vi "ModelProject_backup.vi"() -> ()   [LabVIEW 2011]
uses:
  <vilib>/Simulation/Scripting/Companion Diagram/SimConfigNode/SimParams.ctl
  <vilib>/Simulation/Scripting/Companion Diagram/SimConfigNode/_simSolvers.ctl
  <vilib>/Simulation/Implementation/Shared/SIMSCR Execution Mode.ctl
  <vilib>/Simulation/Param Hierarchy/Typedefs/SIMPH Param Control Actions.ctl
  <vilib>/Simulation/Implementation/Shared/SIM limit type.ctl
  <vilib>/Simulation/Implementation/Shared/NILVSim_FinalizeModel.vi
  <vilib>/Simulation/SignalDisplay/Implementation/NILVSim Buffer XY Graph.llb/SIM Buffer XY Graph (scalar).vi
  <vilib>/Simulation/Utility/Implementation/SIM Time.vi
  <vilib>/Simulation/SignalDisplay/Implementation/NILVSim Time Waveform.llb/SIM Time Waveform (scalar).vi
  <vilib>/Simulation/ContinuousLinear/Implementation/NILVSim Integrator new.llb/SIM Integrator distributor (scalar).vi
  <vilib>/Simulation/ContinuousLinear/Implementation/NILVSim Integrator new.llb/SIM Integrator collector (scalar).vi
  <vilib>/Simulation/ContinuousLinear/Implementation/NILVSim Transfer Function.llb/SIM Transfer Function Collector (SISO).vi
  <vilib>/Simulation/ContinuousLinear/Implementation/NILVSim Transfer Function.llb/SIM Transfer Function Distributor (SISO).vi
  <vilib>/Simulation/ContinuousLinear/Implementation/NILVSim State Space.llb/SIM State Space Distributor (SISO CD).vi
  <vilib>/Simulation/ContinuousLinear/Implementation/NILVSim State Space.llb/SIM State Space Collector (SISO CD).vi
  <vilib>/Simulation/Implementation/Shared/SIM Is Init or Final Stage.vi
  <vilib>/Simulation/Implementation/Shared/NILVSim_Manager.vi
  <vilib>/Simulation/Implementation/Shared/NILVSim_ParamChanged.vi
  <vilib>/Simulation/SignalDisplay/Implementation/NILVSim Buffer XY Graph.llb/NILVSim Buffer XY Graph (core).vi
  <vilib>/Simulation/Implementation/Shared/SIM manage modulo counter.vi
  <vilib>/Simulation/Implementation/Shared/SIM Circular Buffer.llb/SIM CircBuf remove oldest.vi
  <vilib>/Simulation/Implementation/Shared/SIM Circular Buffer.llb/SIM circular buffer insert.vi
  <vilib>/Simulation/Utility/Implementation/NILVSim Get Time and IsAcceptedStep.vi
  <vilib>/addons/Control Design/_Model Construction/Model Creation.llb/Model Creation SubVI/cd_Create State Space Model.vi
  <vilib>/Simulation/Implementation/Shared/SIM Unbundle Sim Info.vi
  <vilib>/Simulation/Implementation/Shared/NILVSim_GetModelError.vi
  <vilib>/Simulation/Implementation/Shared/SIM Bundle Sim Info.vi
  <vilib>/Simulation/Implementation/Shared/NILVSim_Initialize.vi
  SubVI/Poles_Placement.vi
  SubVI/3DMotion.vi
  <vilib>/Analysis/baseanly.llb/Dot Product.vi
  <vilib>/Analysis/baseanly.llb/Real Dot Product.vi
  <vilib>/Simulation/Implementation/Shared/SIM Circular Buffer.llb/SIM circular buffer ordered array.vi
  <vilib>/Simulation/Implementation/Shared/SIM Circular Buffer.llb/SIM circular buffer create.vi
  <vilib>/Simulation/Scripting/Companion Diagram/SimConfigNode/SimDog.xnode
  <vilib>/Simulation/Implementation/XNodeFramework/SimXNode/SimX.xnode
  <vilib>/addons/Control Design/_Model Construction/Model Typedefs.llb/CD General Elements.ctl
  <vilib>/addons/Control Design/_Model Construction/NI_LinSys_Model Typedefs.lvlib
  <vilib>/addons/Control Design/_Model Construction/Model Typedefs.llb/CD State Space Model (MIMO).ctl
  <vilib>/Analysis/NI_AALBase.lvlib
  <vilib>/Simulation/ContinuousLinear/Implementation/NILVSim State Space.llb/SIM State Space (SISO CD).vi
  <vilib>/Simulation/ContinuousLinear/Implementation/NILVSim Transfer Function.llb/SIM Transfer Function (SISO).vi
  <vilib>/addons/Control Design/_Model Construction/NI_LinSys_Model Creation.lvlib
  <vilib>/Simulation/ContinuousLinear/Implementation/NILVSim Integrator new.llb/SIM Integrator (scalar).vi
  <vilib>/Simulation/Implementation/Shared/NI_SIM_Implementation.lvlib
panel:
  in  "Z -ALT":dbl(slide)=50.0 scale=0.0..1000.0
  in  "PSI":dbl(slide) scale=-170.0..170.0
  in  "Theta":dbl(slide) scale=-45.0..45.0
  in  "PHAI":dbl(slide) scale=-45.0..45.0
  out "X":waveform(dbl)(graph)={"t0"=timestamp(9343.2 s since 1904-01-01), "dt"=1.0, "Y"=[0.2633720690985406]}
  out "Y":waveform(dbl)(graph)={"t0"=timestamp(9343.2 s since 1904-01-01), "dt"=1.0, "Y"=[0.2633720690985406]}
  out "Time (sec)":dbl
  out "Y_Process":dbl
  out "X_Process":dbl
  out "SPEED":dbl(knob) scale=1.0..1000.0
  in  "RESET":bool
  in  "STOP":bool
  out "STOP":bool
  out "RUN":bool
  out "uZ":dbl(graph)
  out "uPHAI":dbl(graph)
  out "uTH":dbl(graph)
  out "uPSI":dbl(graph)
  out "PHAI":dbl(graph)
  out "Z graph":dbl(graph)
  out "THETA":dbl(graph)
  out "XY Graph":cluster{"X":dbl, "Y":dbl}[](graph)
  out "W4":dbl(knob) scale=0.0..10000.0
  out "W3":dbl(knob) scale=0.0..10000.0
  out "W2":dbl(knob) scale=0.0..10000.0
  out "W1":dbl(knob) scale=0.0..10000.0
  out "PSI":dbl(graph)
  out "uZ(k)":dbl(slide) scale=0.0..1.0 scale format="%.2p"
  out "Controllers PSI 5":enum32{"Page 1", "Page 2"}(tab)
  out "Z Desired Poles":cdb[](array[numeric])=[-4.951252167649562+0.0i, -3.4076115316471642-10.013861291935129i, -3.4076115316471642+10.013861291935129i] format="%.2f"
  in  "Real Z":dbl(knob)=-3.4076115316471642 scale=0.0..-22.0 scale format="%#_4g"
  out "Z Actual Poles":cdb[](array[numeric])=[-4.9512521676495505+0.0i, -3.4076115316471447-10.013861291935113i, -3.4076115316471447+10.013861291935113i] format="%.2f"
  out "Gain Z":dbl[](array[numeric])
  out "state xZ(k)":dbl[](array[numeric])
  in  "Zdot":dbl(slide)=1.0 scale=0.0..10.0
  in  "Imaginary Z":dbl(knob) scale=0.0..10.0
  out "Z Closed-Loop Step Response":cluster{"time":dbl[], dbl[]}[](graph)
  out "Z State Trajectory Graph":cluster{"time":dbl[], dbl[]}[](graph)
  out "Z":dbl(slide)=100.0 scale=0.0..1000.0
  out "uph(k)":dbl(slide) scale=0.0..0.5 scale format="%.2p"
  out "Controllers PSI 4":enum32{"Page 1", "Page 2"}(tab)
  out "Phi Desired Poles":cdb[](array[numeric])=[-4.951252167649562+0.0i, -3.4076115316471642-10.013861291935129i, -3.4076115316471642+10.013861291935129i] format="%.2f"
  in  "Real Phi":dbl(knob)=-3.4076115316471642 scale=0.0..-22.0 scale format="%#_4g"
  out "Phi Actual Poles":cdb[](array[numeric])=[-4.9512521676495505+0.0i, -3.4076115316471447-10.013861291935113i, -3.4076115316471447+10.013861291935113i] format="%.2f"
  out "Phi":dbl(slide)=1.0 scale=-45.0..45.0
  out "Gain Phi":dbl[](array[numeric])
  out "state xphi(k)":dbl[](array[numeric])
  in  "Phidot":dbl(slide)=1.0 scale=0.0..10.0
  in  "Imaginary Phi":dbl(knob) scale=0.0..10.0
  out "Phi Closed-Loop Step Response":cluster{"time":dbl[], dbl[]}[](graph)
  out "Phi State Trajectory Graph":cluster{"time":dbl[], dbl[]}[](graph)
  out "uth(k)":dbl(slide) scale=0.0..1.0 scale format="%.2p"
  out "Controllers PSI 3":enum32{"Page 1", "Page 2"}(tab)
  out "Th Desired Poles":cdb[](array[numeric])=[-4.951252167649562+0.0i, -3.4076115316471642-10.013861291935129i, -3.4076115316471642+10.013861291935129i] format="%.2f"
  in  "Real Th":dbl(knob)=-3.4076115316471642 scale=0.0..-22.0 scale format="%#_4g"
  out "Th Actual Poles":cdb[](array[numeric])=[-4.9512521676495505+0.0i, -3.4076115316471447-10.013861291935113i, -3.4076115316471447+10.013861291935113i] format="%.2f"
  out "Theta":dbl(slide)=1.0 scale=-45.0..45.0
  out "Gain Th":dbl[](array[numeric])
  out "state xth(k)":dbl[](array[numeric])
  in  "Thdot":dbl(slide)=1.0 scale=0.0..10.0
  in  "Imaginary Th":dbl(knob) scale=0.0..10.0
  out "Th Closed-Loop Step Response":cluster{"time":dbl[], dbl[]}[](graph)
  out "Th State Trajectory Graph":cluster{"time":dbl[], dbl[]}[](graph)
  out "upsi(k)":dbl(slide) scale=0.0..0.5 scale format="%.2p"
  out "Controllers PSI":enum32{"Page 1", "Page 2"}(tab)
  out "Psi Desired Poles":cdb[](array[numeric])=[-4.951252167649562+0.0i, -3.4076115316471642-10.013861291935129i, -3.4076115316471642+10.013861291935129i] format="%.2f"
  in  "Real Psi":dbl(knob)=-3.4076115316471642 scale=0.0..-22.0 scale format="%#_4g"
  out "Psi Actual Poles":cdb[](array[numeric])=[-4.9512521676495505+0.0i, -3.4076115316471447-10.013861291935113i, -3.4076115316471447+10.013861291935113i] format="%.2f"
  out "Psi":dbl(slide)=1.0 scale=-180.0..180.0
  out "Gain Psi":dbl[](array[numeric])
  out "state xpsi(k)":dbl[](array[numeric])
  in  "Psidot":dbl(slide)=1.0 scale=0.0..10.0
  in  "Imaginary Psi":dbl(knob) scale=0.0..10.0
  out "Psi Closed-Loop Step Response":cluster{"time":dbl[], dbl[]}[](graph)
  out "Psi State Trajectory Graph":cluster{"time":dbl[], dbl[]}[](graph)
  in  "name or relative path":string="..\\Hexa1.stl"
  out "3D path":path
  out "3D Picture Control":refnum<vi>(3d-picture)
  out "PSI (k) deg":dbl
  out "THETA (k) deg":dbl
  out "PHAI (k) deg":dbl
  out "Z (k) m":dbl
  # "Feedback PSI"
  # "Feedback THETA"
  # "Feedback PHAI"
  # "y(k)"
  # "Gains\n           k0, k1"
  # "Quadcopter"
  # "e1(k)"
  # "uz(k)"
  # "uphi(k)"
  # "e2(k)"
  # "Gains\n           k2, k3"
  # "x0\nx1\n\nx2\nx3\n\nx4\nx5\n\nx6\nx7"
  # "Gains\n           k4, k5"
  # "e3(k)"
  # "uth(k)"
  # "Gains\n           k6, k7"
  # "e4(k)"
  # "upsi(k)"
  # "Feedback Z"
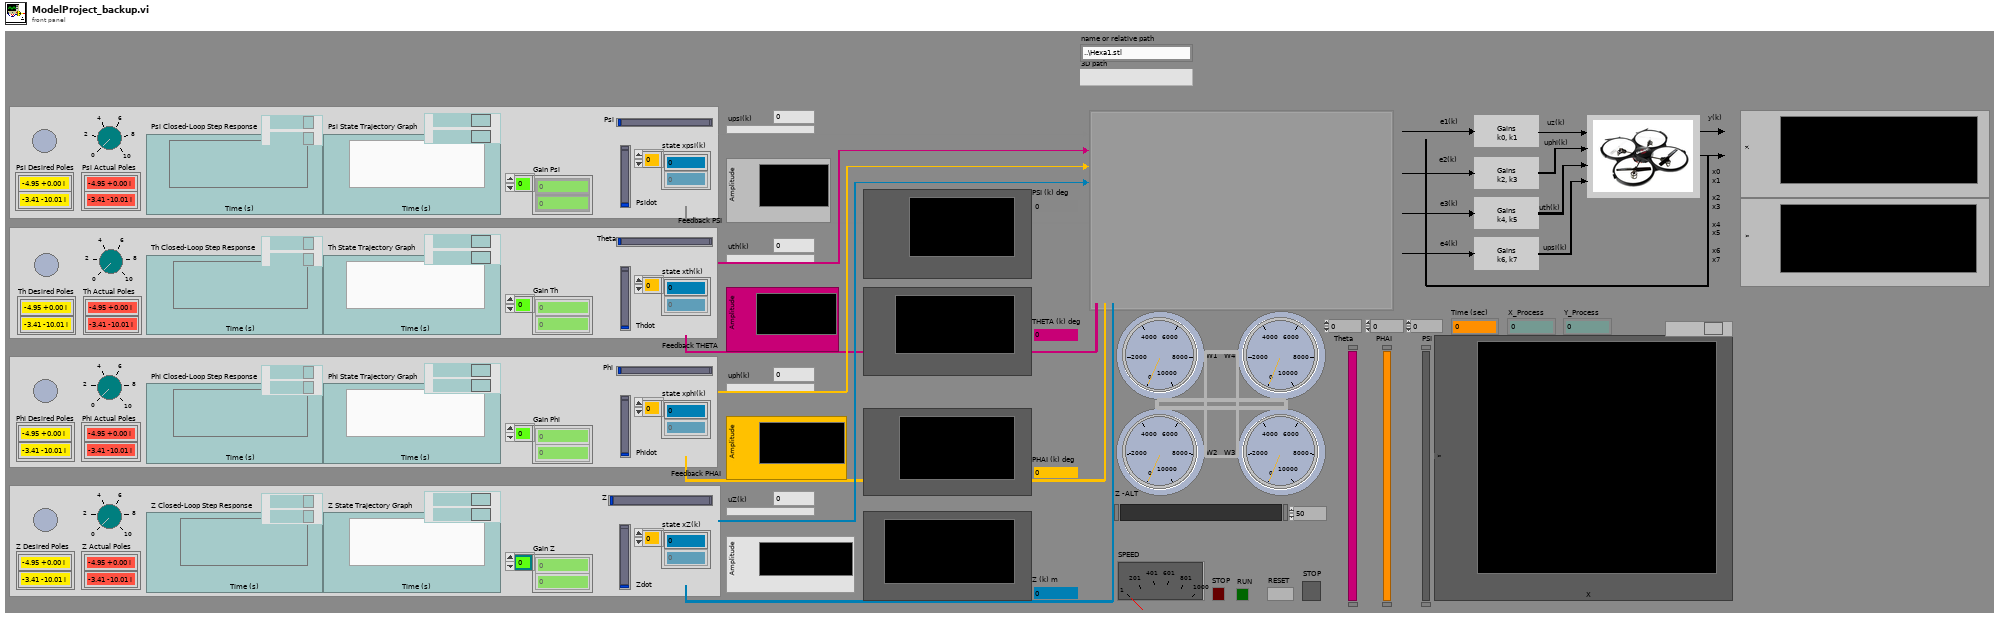
[diagram p1: front panel]
types:
  T1 = typedef "NI_LinSys_Model Typedefs.lvlib/CD State Space Model (MIMO).ctl" = cluster{"properties":T2, "A":dbl[][], "B":dbl[][], "C":dbl[][], "D":dbl[][], "StateNames":string[], "Transport Delay":dbl[][]}
  T2 = typedef "NI_LinSys_Model Typedefs.lvlib/CD General Elements.ctl" = cluster{"Model name":string, "Input names":string[], "Output names":string[], "Input Delays":dbl[], "Output Delays":dbl[], "Sampling Time":dbl, "Notes":string}
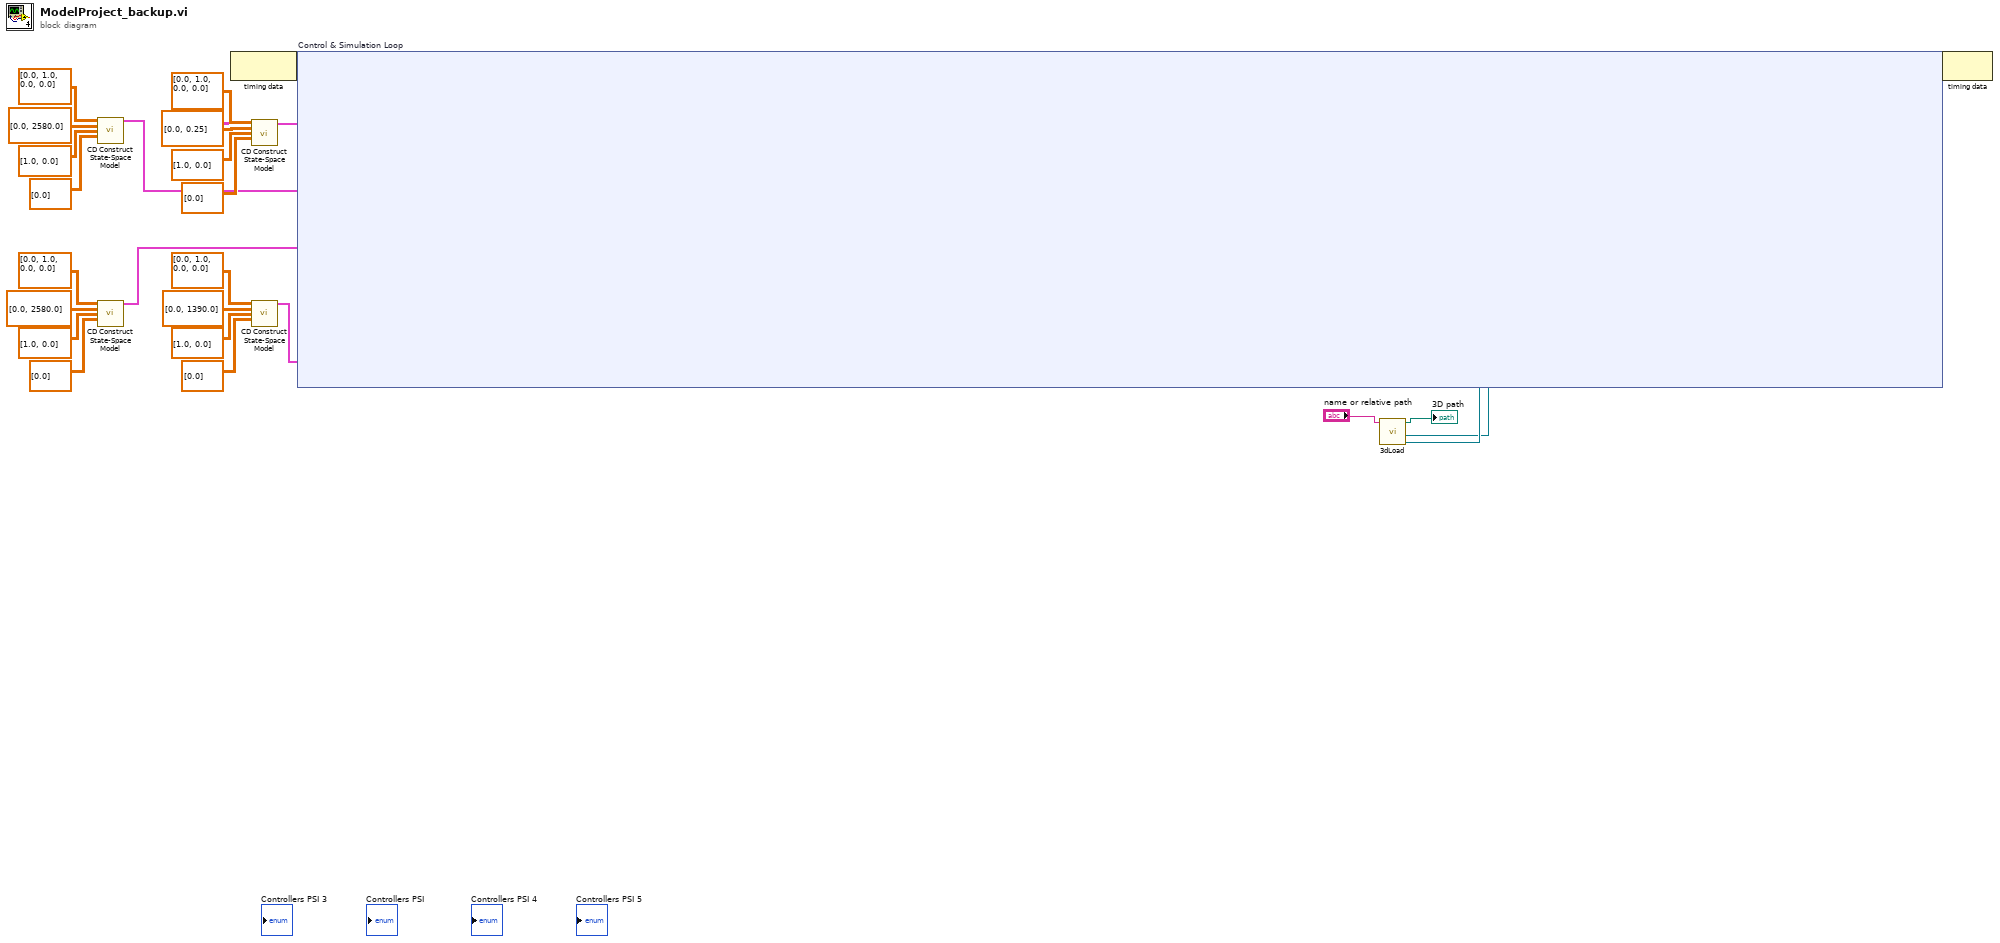
[diagram p0: block diagram]
diagram:
  n1 = call-poly <vilib>:"CD Construct State-Space Model.vi"("A"=dbl[][] [[0.0, 1.0], [0.0, 0.0]], "B"=dbl[][] [[0.0], [2580.0]], "C"=dbl[][] [[1.0, 0.0]], "D"=dbl[][] [[0.0]]) -> ("State-Space Model"=w6:T1)  [unwired: 10 in, 1 out]
  n2 = call-poly <vilib>:"CD Construct State-Space Model.vi"("A"=dbl[][] [[0.0, 1.0], [0.0, 0.0]], "B"=dbl[][] [[0.0], [2580.0]], "C"=dbl[][] [[1.0, 0.0]], "D"=dbl[][] [[0.0]]) -> ("State-Space Model"=w7:T1)  [unwired: 10 in, 1 out]
  n3 = node-c288() -> (w26:variant)  [unwired: 1 in]
  n4 = call-poly <vilib>:"CD Construct State-Space Model.vi"("A"=dbl[][] [[0.0, 1.0], [0.0, 0.0]], "B"=dbl[][] [[0.0], [0.25]], "C"=dbl[][] [[1.0, 0.0]], "D"=dbl[][] [[0.0]]) -> ("State-Space Model"=w20:T1)  [unwired: 10 in, 1 out]
  n5 = call-poly <vilib>:"CD Construct State-Space Model.vi"("A"=dbl[][] [[0.0, 1.0], [0.0, 0.0]], "B"=dbl[][] [[0.0], [1390.0]], "C"=dbl[][] [[1.0, 0.0]], "D"=dbl[][] [[0.0]]) -> ("State-Space Model"=w5:T1)  [unwired: 10 in, 1 out]
  n6 = call "3dLoad.vi"("name or relative path"="name or relative path") -> ("Object"=w2:refnum<vi>, "reference out"=w1:refnum<vi>, "appended path 2"=→"3D path":path)  [unwired: 8 in]
  n7 = node-c254 "Control & Simulation Loop"(w26, w20, w7, w6, w5, w2, w1) -> (w25:variant)
  n8 = node-c288(w25) -> ()  [unwired: 1 out]
